vi "Wave1D_Init Sol.vi"(10 "Boundary Condition":cluster{"type":T2, "Value":dbl[]}[](array[cluster]) {"type" items=["Dirichlet", "Neumann"]}, 11 "Domain":T1={"t"={"initial t"=0.0, "final t"=1.0, "# of t-points"=11}, "x"={"start x"=0.0, "end x"=1.0, "# of x-points"=11}}) -> (3 "U(t, x)":dbl[][](array[numeric]))   [LabVIEW 2017, in "NI_PDE.lvlib"]
uses:
  <vilib>/gmath/NI_PDE.lvlib
  <vilib>/gmath/pde.llb/Common/PDE_BC Type.ctl
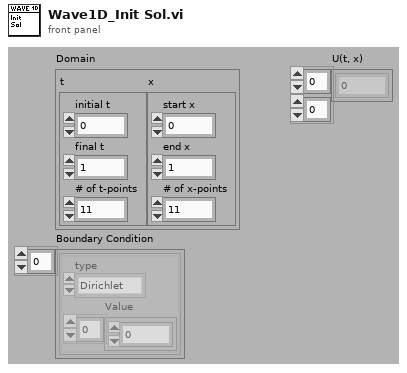
[diagram p1: front panel]
types:
  T1 = cluster{"t":cluster{"initial t":dbl, "final t":dbl, "# of t-points":i32}, "x":cluster{"start x":dbl, "end x":dbl, "# of x-points":i32}}
  T2 = typedef "NI_PDE.lvlib/PDE_BC Type.ctl" = i32
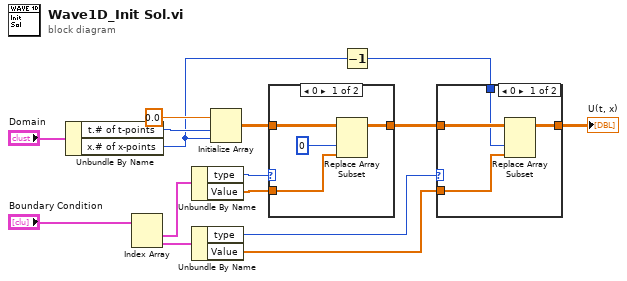
[diagram p0: block diagram]
diagram:
  n1 = Unbundle By Name("Domain") -> ("t.# of t-points"=w10:i32, "x.# of x-points"=w2:i32)
  n2 = Index Array(array="Boundary Condition") -> (element #1=w14:cluster{"type":T2, "Value":dbl[]}, element #2=w13:cluster{"type":T2, "Value":dbl[]})  [unwired: 2 in]
  n3 = Unbundle By Name(w14) -> ("type"=w9:T2, "Value"=w7:dbl[])
  n4 = Unbundle By Name(w13) -> ("type"=w5:T2, "Value"=w4:dbl[])
  n5 = Initialize Array(0.0 ("element"), w10, w2) -> (w8:dbl[][])
  n6 = case shown="0" w9 {
    tunnel: w8 -> [w19 w20]
    tunnel: w7 -> [w17 _]
    tunnel: [w16 w20] -> w6
    frame 0 {
      n7 = Replace Array Subset(array=w19, new element=w17, index (col)=0 ("disabled index (col)")) -> (w16:dbl[][])  [unwired: 1 in]
    }
    frame 1, Default {
    }
  }
  n8 = Decrement(x=w2) -> (x-1=w1:i32)
  n9 = case shown="0" w5 {
    tunnel: w6 -> [w24 w25]
    tunnel: w4 -> [w23 _]
    tunnel: [w22 w25] -> w3
    tunnel: w1 -> [w21 _]
    frame 0 {
      n10 = Replace Array Subset(array=w24, new element=w23, index (col)=w21) -> (w22:dbl[][])  [unwired: 1 in]
    }
    frame 1, Default {
    }
  }
  "U(t, x)" <- w3
